vi "BeadCoolerFixedZ(SubVI)_extraHP.vi"(1 "AI0":i16, 2 "Dc Pos":i16, 5 "ig":fxp<+/-,24,6>, 7 "dg":fxp<+/-,24,12>, 8 "hp coeff":i32[](array[numeric])=[946630756, 1010186290], 9 "pg":fxp<+/-,24,12>, 11 "Use highpass":bool, 12 "lp coeff":i32[](array[numeric])=[1008310688, 32715568], 13 "Upper lim":fxp<+/-,16,16>, 14 "Lower lim":fxp<+/-,16,16>, 15 "hp coeff 2":i32[](array[numeric])=[-898916953, 1957103775, 982440638]) -> (10 "Output":fxp<+/-,16,16>)   [LabVIEW 2013]
uses:
  <vilib>/rvi/FXPMathLib/basic elements/FxpIntAccumulator/subVIs/nifxpmath_IntAccumulator_SimConfig.ctl
  <vilib>/rvi/FXPMathLib/basic elements/FxpIntAccumulator/simVIs/DllFxpIntAccumulator_sub.vi
  <vilib>/rvi/FXPMathLib/FxpInterpret/XNode/nifxpmath_Interpret.xnode
  <vilib>/rvi/Analysis/measure/butterworth/XNode/niFpgaButterworthFilter.xnode
  <vilib>/rvi/FXPMathLib/basic elements/FxpIntAccumulator/XNode/nifxpmath_IntAccumulator.xnode
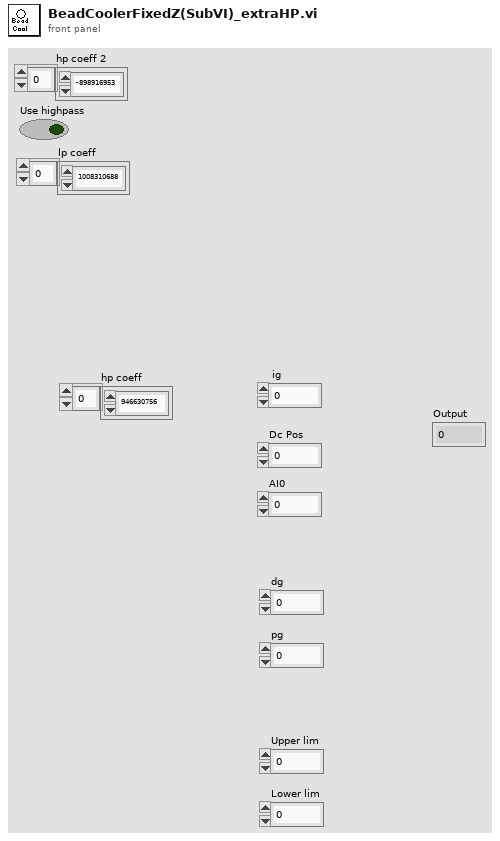
[diagram p1: front panel]
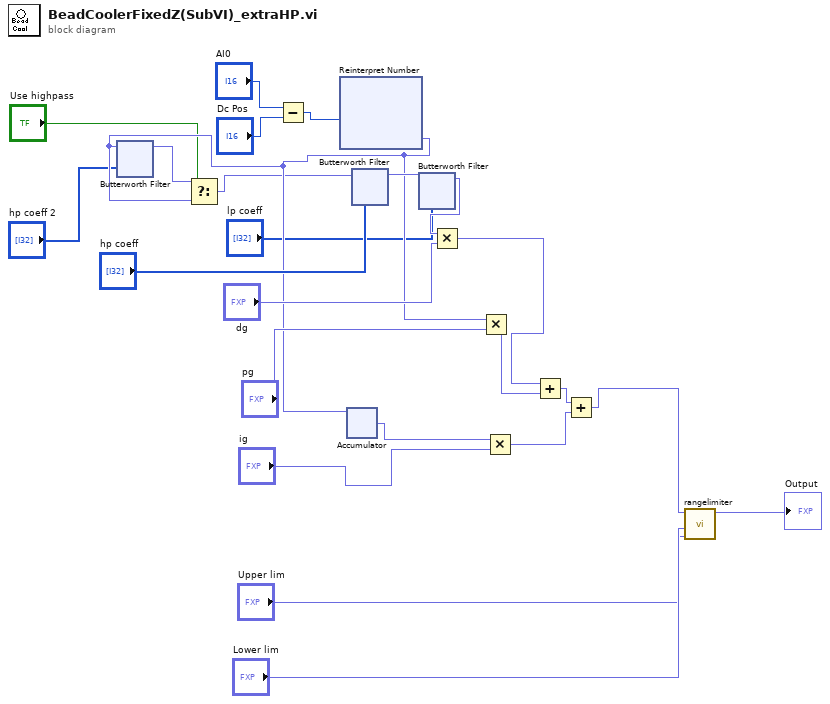
[diagram p0: block diagram]
diagram:
  n1 = Subtract(x="AI0", y="Dc Pos") -> (x-y=w18:i16)
  n2 = xnode "Reinterpret Number"("x"=w18) -> ("y"=w5:fxp<+/-,16,16>)
  n3 = xnode "Butterworth Filter"("input data"=w5, "scaled coefficients"="hp coeff 2") -> ("output data"=w6:fxp<+/-,20,20>)  [unwired: 1 in]
  n4 = Select(t=w6, s="Use highpass", f=w5) -> (s? t:f=w4:fxp<+/-,20,20>)
  n5 = xnode "Accumulator"("x"=w5) -> ("s"=w11:fxp<+/-,32,32>)  [unwired: 4 in, 1 out]
  n6 = xnode "Butterworth Filter"("input data"=w4, "scaled coefficients"="hp coeff") -> ("output data"=w9:fxp<+/-,24,24>)  [unwired: 1 in]
  n7 = xnode "Butterworth Filter"("input data"=w9, "scaled coefficients"="lp coeff") -> ("output data"=w8:fxp<+/-,28,28>)  [unwired: 1 in]
  n8 = Multiply(x=w8, y="dg") -> (x*y=w7:fxp<+/-,24,23>)
  n9 = Multiply(x=w5, y="pg") -> (x*y=w24:fxp<+/-,24,23>)
  n10 = Multiply(x=w11, y="ig") -> (x*y=w13:fxp<+/-,24,23>)
  n11 = Add(x=w7, y=w24) -> (x+y=w15:fxp<+/-,24,23>)
  n12 = Add(x=w15, y=w13) -> (x+y=w14:fxp<+/-,16,16>)
  n13 = call "rangelimiter.vi"("Upper lim"="Upper lim", "Lower lim"="Lower lim", "Input"=w14) -> ("Output"=→"Output":fxp<+/-,16,16>)  [unwired: 8 in]
